vi "Seed&key算法.vi"(1 "解锁类型":enum16{"读取", "写", "下载"}(ring), 2 "Seed":u32[](array[numeric]) format="%x") -> (0 "key":u32)   [LabVIEW 2013]
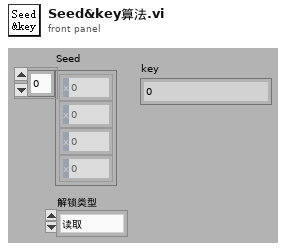
[diagram p1: front panel]
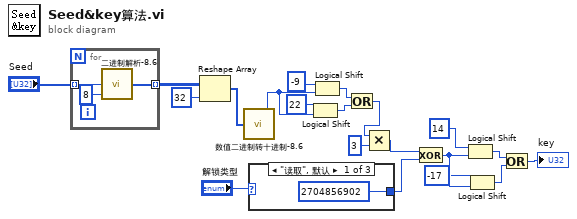
[diagram p0: block diagram]
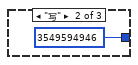
[diagram p2: hidden frame]
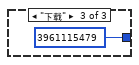
[diagram p3: hidden frame]
diagram:
  n1 = for {
    tunnel: "Seed" -> [w23] mode=indexing
    tunnel: [w21] -> w20 mode=indexing
    n2 = call "二进制解析-8.6.vi"("索引"=8, "数值"=w23) -> ("低位子数组"=w21:i32[])  [unwired: 3 out]
  }
  n3 = Reshape Array(w20, u32 32 ("维数大小")) -> (w18:i32[])
  n4 = call "数值二进制转十进制-8.6.vi"("子数组"=w18) -> ("十进制数值"=w5:i32)  [unwired: 4 out]
  n5 = case shown="\"读取\", 默认" "解锁类型" {
    tunnel: [u32 2704856902 ("y") u32 3549594946 ("y") u32 3961115479 ("y")] -> w12
    frame "读取", Default {
    }
    frame "写" {
    }
    frame "下载" {
    }
  }
  n6 = Logical Shift(y=22, x=w5) -> (x << y=w2:i32)
  n7 = Logical Shift(y=-9, x=w5) -> (x << y=w3:i32)
  n8 = Or(x=w3, y=w2) -> (x .or. y?=w1:i32)
  n9 = Multiply(x=w1, y=u32 3) -> (x*y=w14:u32)
  n10 = Exclusive Or(1:w12, 2:w14) -> (0:w10:u32)
  n11 = Logical Shift(y=u32 14, x=w10) -> (x << y=w8:u32)
  n12 = Logical Shift(y=-17, x=w10) -> (x << y=w7:u32)
  n13 = Or(x=w8, y=w7) -> (x .or. y?=→"key":u32)
